vi "TAT_Com_PLC.vi"() -> ()   [LabVIEW 2017]
uses:
  <vilib>/NI/Modbus Library/API/Wrapper/Create TCP Master.vi
  Global/Global 1.vi
  <vilib>/NI/Modbus Library/API/Master/Modbus Master.lvclass
  <vilib>/NI/Modbus Library/API/Wrapper/API Main.lvlib
panel:
  out "Write to PLC":bool[](array[boolean])
  out "error out":errorcluster
  out "Read From PLC":u16[](array[numeric])
  out "PLC STATUS":bool
  in  "error in":errorcluster
  in  "stop":bool
  # "Ass & Leak"
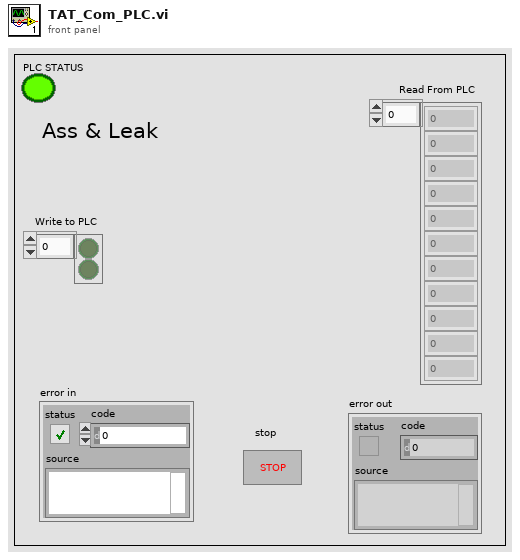
[diagram p1: front panel]
types:
  T1 = enum32{"invalid app kind", "Development System", "Run Time System", "Student Edition", "Embedded LabVIEW", "Evaluation", "Custom"}
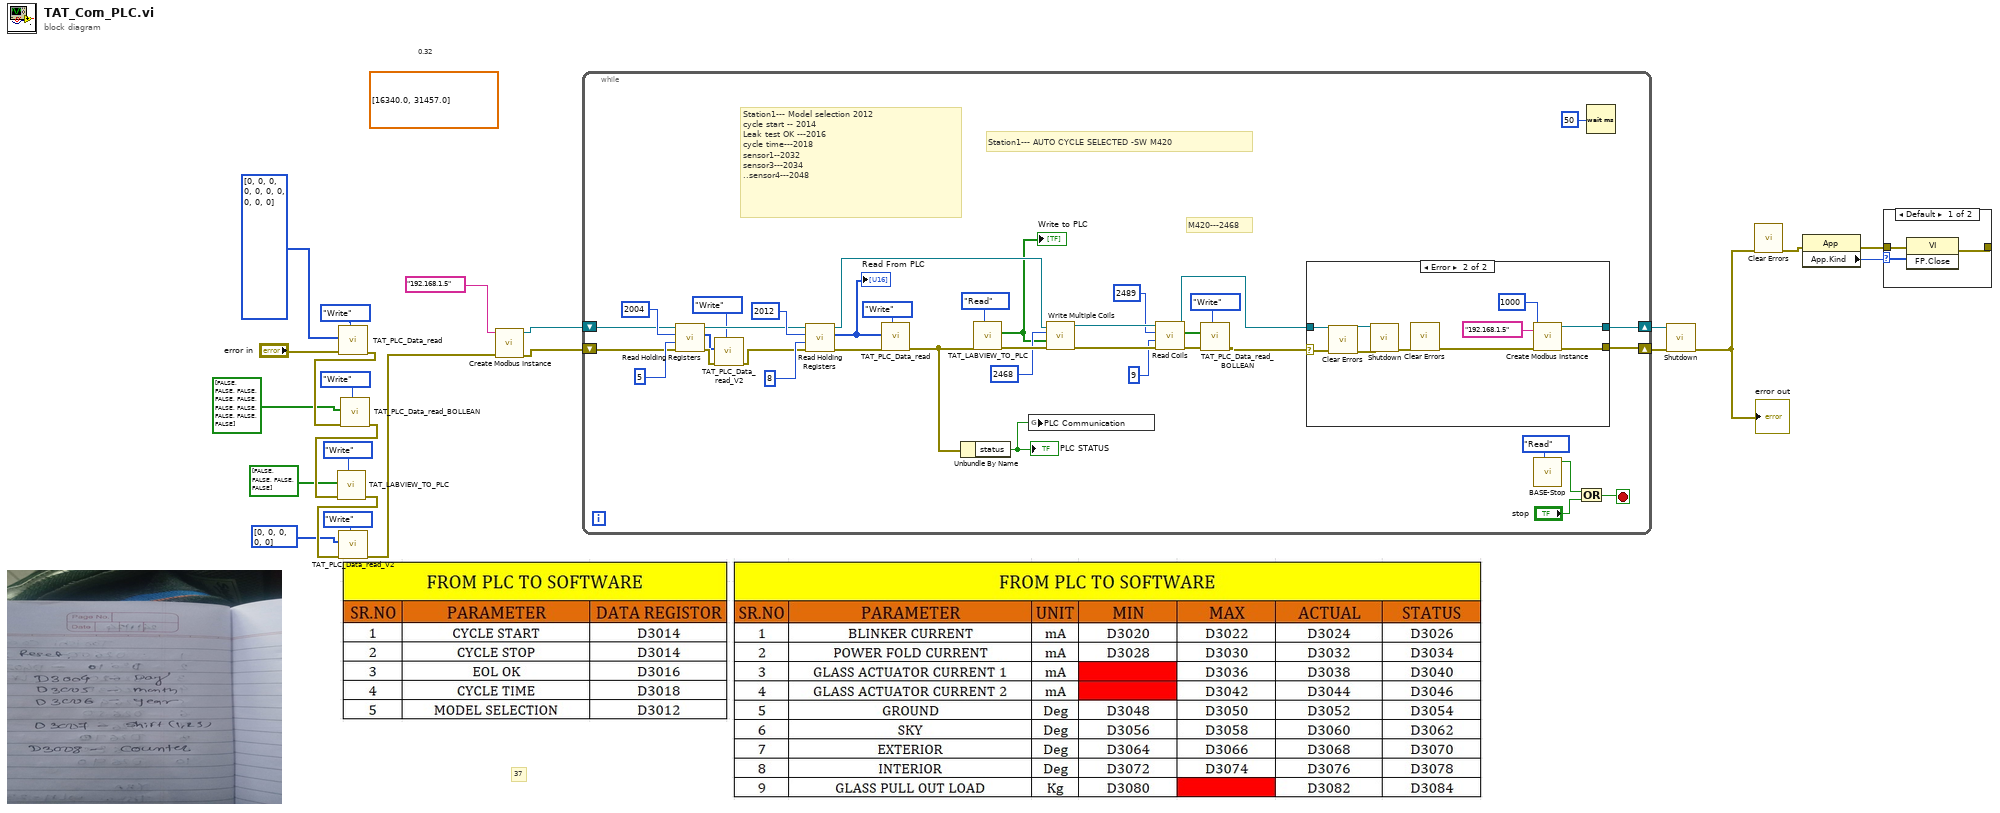
[diagram p0: block diagram]
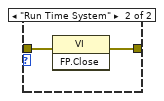
[diagram p3: hidden frame]
diagram:
  (unwired) dbl[] [16340.0, 31457.0] ("register values")
  # "37"
  # "0.32"
  n1 = call "TAT_PLC_Data_read.vi"("Enum"=enum16{"Read", "Write"}."Write", "error in (no error)"="error in", "Array"=i64[] [0, 0, 0, 0, 0, 0, 0, 0, 0, 0] ("Array 3")) -> ("error out"=w11:errorcluster)  [unwired: 7 in, 1 out]
  n2 = call "TAT_PLC_Data_read_BOLLEAN.vi"("Enum"=enum16{"Read", "Write"}."Write", "error in (no error)"=w11, "Array"=bool[] [FALSE, FALSE, FALSE, FALSE, FALSE, FALSE, FALSE, FALSE, FALSE, FALSE]) -> ("error out"=w8:errorcluster)  [unwired: 7 in, 1 out]
  n3 = call "TAT_LABVIEW_TO_PLC.vi"("Enum"=enum16{"Read", "Write"}."Write", "error in (no error)"=w8, "Array"=bool[] [FALSE, FALSE, FALSE, FALSE]) -> ("error out"=w3:errorcluster)  [unwired: 7 in, 1 out]
  n4 = call "TAT_PLC_Data_read_V2.vi"("Enum"=enum16{"Read", "Write"}."Write", "error in (no error)"=w3, "Array"=u16[] [0, 0, 0, 0, 0] ("Array 3")) -> ("error out"=w2:errorcluster)  [unwired: 7 in, 1 out]
  n5 = call-poly <vilib>:"Create Modbus Instance.vi"("error in"=w2, "address"="192.168.1.5") -> ("error out"=w17:errorcluster, "TCP master instance"=w16:refnum<class "Modbus Master.lvclass">)  [unwired: 8 in]
  n6 = while {
    shift-right: [w57] -> w21
    shift-left: w16 -> [w29]
    shift-right: [w56] -> w20
    shift-left: w17 -> [w27]
    stop <- w58 stop-if-true
    # "M420---2468"
    # "Station1--- AUTO CYCLE SELECTED -SW M420"
    # "Station1--- Model selection 2012\ncycle start -- 2014\nLeak test OK ---2016\ncycle time---2018\nsensor1--2032\nsensor3---2034\n..sensor4---2048"
    n7 = call-dynamic "Read Holding Registers.vi"("error in"=w27, "number of inputs"=u16 5, "starting address"=u16 2004, "Modbus master in"=w29) -> ("error out"=w26:errorcluster, "register values"=w24:u16[], "Modbus master out"=w28:refnum<class "Modbus Master.lvclass">)  [unwired: 5 in]
    n8 = call "TAT_PLC_Data_read_V2.vi"("Enum"=enum16{"Read", "Write"}."Write", "error in (no error)"=w26, "Array"=w24) -> ("error out"=w25:errorcluster)  [unwired: 7 in, 1 out]
    n9 = call-dynamic "Read Holding Registers.vi"("error in"=w25, "number of inputs"=u16 8, "starting address"=u16 2012, "Modbus master in"=w28) -> ("error out"=w51:errorcluster, "register values"=w43:u16[], "Modbus master out"=w49:refnum<class "Modbus Master.lvclass">)  [unwired: 5 in]
    "Read From PLC" <- w43
    n10 = call "TAT_PLC_Data_read.vi"("Enum"=enum16{"Read", "Write"}."Write", "error in (no error)"=w51, "Array"=w43) -> ("error out"=w50:errorcluster)  [unwired: 7 in, 1 out]
    n11 = Unbundle By Name(w50) -> ("status"=w32:bool)
    "PLC STATUS" <- w32
    n12 = call "TAT_LABVIEW_TO_PLC.vi"("Enum"=enum16{"Read", "Write"}."Read", "error in (no error)"=w50) -> ("error out"=w47:errorcluster, "Array 2"=w42:bool[])  [unwired: 8 in]
    "Write to PLC" <- w42
    n13 = global write "Global 1.vi" "PLC Communication"(w32) -> ()
    n14 = call-dynamic "Write Multiple Coils.vi"("error in"=w47, "coils to write"=w42, "starting address"=u16 2468, "Modbus master in"=w49) -> ("error out"=w40:errorcluster, "Modbus master out"=w39:refnum<class "Modbus Master.lvclass">)  [unwired: 6 in]
    n15 = call-dynamic "Read Coils.vi"("error in"=w40, "number of inputs"=u16 9, "starting address"=u16 2489, "Modbus master in"=w39) -> ("error out"=w34:errorcluster, "coils"=w35:bool[], "Modbus master out"=w38:refnum<class "Modbus Master.lvclass">)  [unwired: 5 in]
    n16 = call "TAT_PLC_Data_read_BOLLEAN.vi"("Enum"=enum16{"Read", "Write"}."Write", "error in (no error)"=w34, "Array"=w35) -> ("error out"=w33:errorcluster)  [unwired: 7 in, 1 out]
    n17 = case shown="Error" w33 {
      selector: w33 -> [w60 w70]
      tunnel: w38 -> [w61 w68]
      tunnel: [w61 w64] -> w57
      tunnel: [w60 w63] -> w56
      frame No Error {
      }
      frame Error {
        n18 = call <vilib>:"Clear Errors.vi"("error in (no error)"=w70) -> ("error out"=w69:errorcluster)  [unwired: 5 in, 1 out]
        n19 = call-dynamic "Shutdown.vi"("error in"=w69, "Modbus master in"=w68) -> ("error out"=w67:errorcluster)  [unwired: 9 in]
        n20 = call <vilib>:"Clear Errors.vi"("error in (no error)"=w67) -> ("error out"=w65:errorcluster)  [unwired: 5 in, 1 out]
        n21 = call-poly <vilib>:"Create Modbus Instance.vi"("error in"=w65, "connect timeout ms"=1000, "address"="192.168.1.5") -> ("error out"=w63:errorcluster, "TCP master instance"=w64:refnum<class "Modbus Master.lvclass">)  [unwired: 7 in]
      }
    }
    n22 = call "BASE-Stop.vi"("Enum"=enum16{"Read", "Write"}."Read") -> ("Stop"=w44:bool)  [unwired: 10 in]
    n23 = Or(x=w44, y="stop") -> (x .or. y?=w58:bool)
    n24 = Wait (ms)(milliseconds to wait=u32 50) -> ()  [unwired: 1 out]
  }
  n25 = call-dynamic "Shutdown.vi"("error in"=w20, "Modbus master in"=w21) -> ("error out"=w6:errorcluster)  [unwired: 9 in]
  "error out" <- w6
  n26 = call <vilib>:"Clear Errors.vi"("error in (no error)"=w6) -> ("error out"=w5:errorcluster)  [unwired: 5 in, 1 out]
  n27 = property class="App"(error in=w5) -> (error out=w18:errorcluster, "App.Kind"=w19:T1)  [unwired: 1 in, 1 out]
  n28 = case shown="Default" w19 {
    tunnel: w18 -> [w72 w74]
    tunnel: [w71 w73] -> _
    frame Default {
      n29 = invoke class="VI" method="FP.Close"(error in=w72) -> (error out=w71:errorcluster)  [unwired: 2 in, 2 out]
    }
    frame "Run Time System" {
      n30 = invoke class="VI" method="FP.Close"(error in=w74) -> (error out=w73:errorcluster)  [unwired: 2 in, 2 out]
    }
  }
